vi "Edit Items.vi"(11 "Display State In":T1={"Persistent"={"Elements"=[], "PicElements"=[], "Limits"=[], "Selection"=[], "Selection Color"=0, "Highlight"=[], "Highlight Val"=0, "Highlight Color"={"Back"=0, "Edge"=0}, "Font"={"Details"={"Font Name:"="Lucida Sans", "Size"=24, "Strikeout?"=FALSE, "Italic?"=FALSE, "Underline?"=FALSE, "Outline?"=FALSE, "Shadow?"=FALSE, "Bold?"=TRUE}, "Color"=7697781}, "Bakground Color"=0}, "List Ref"=refnum, "nbVisible"=0, "FirstIdx"=0, "More.Width"=0}) -> (2 "Changed":bool, 3 "Display State out":T1={"Persistent"={"Elements"=[], "PicElements"=[], "Limits"=[], "Selection"=[], "Selection Color"=0, "Highlight"=[], "Highlight Val"=0, "Highlight Color"={"Back"=0, "Edge"=0}, "Font"={"Details"={"Font Name:"="Lucida Sans", "Size"=24, "Strikeout?"=FALSE, "Italic?"=FALSE, "Underline?"=FALSE, "Outline?"=FALSE, "Shadow?"=FALSE, "Bold?"=TRUE}, "Color"=7697781}, "Bakground Color"=0}, "List Ref"=refnum, "nbVisible"=0, "FirstIdx"=0, "More.Width"=0} caption="Display State Out")   [LabVIEW 2016, in "Horizontal MenuList.xctl"]
uses:
  Horizontal MenuList.xctl
  Horizontal MenuList_State.ctl
  Highlight Colors.ctl
  Edit_Actions.ctl
panel:
  out "Stop":bool
  in  "Move Down":bool
  in  "Move Up":bool
  in  "Delete":bool
  in  "Insert":bool
  out "Preview":picture
  in  "Item Pairs":i32(listbox)
  in  "Cancel":bool
  in  "OK":bool
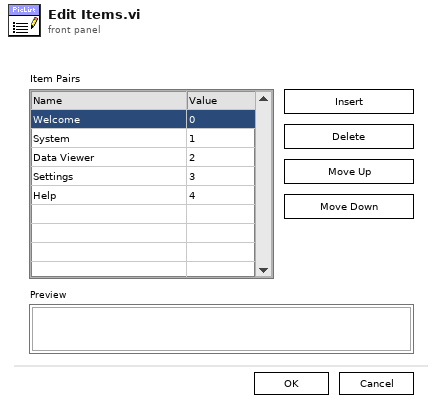
[diagram p1: front panel]
types:
  T1 = typedef "Horizontal MenuList.xctl/Horizontal MenuList_State.ctl" = cluster{"Persistent":cluster{"Elements":string[], "PicElements":picture[], "Limits":i32[], "Selection":picture[], "Selection Color":u32, "Highlight":picture[], "Highlight Val":i32, "Highlight Color":T2, "Font":cluster{"Details":cluster{"Font Name:":string, "Size":i16, "Strikeout?":bool, "Italic?":bool, "Underline?":bool, "Outline?":bool, "Shadow?":bool, "Bold?":bool}, "Color":u32}, "Bakground Color":u32}, "List Ref":refnum<vi>, "nbVisible":u8, "FirstIdx":u8, "More.Width":u8}
  T2 = typedef "Horizontal MenuList.xctl/Highlight Colors.ctl" = cluster{"Back":u32, "Edge":u32}
  T3 = typedef "Horizontal MenuList.xctl/Edit_Actions.ctl" = enum16{"Insert", "Delete", "Move Up", "Move Down"}
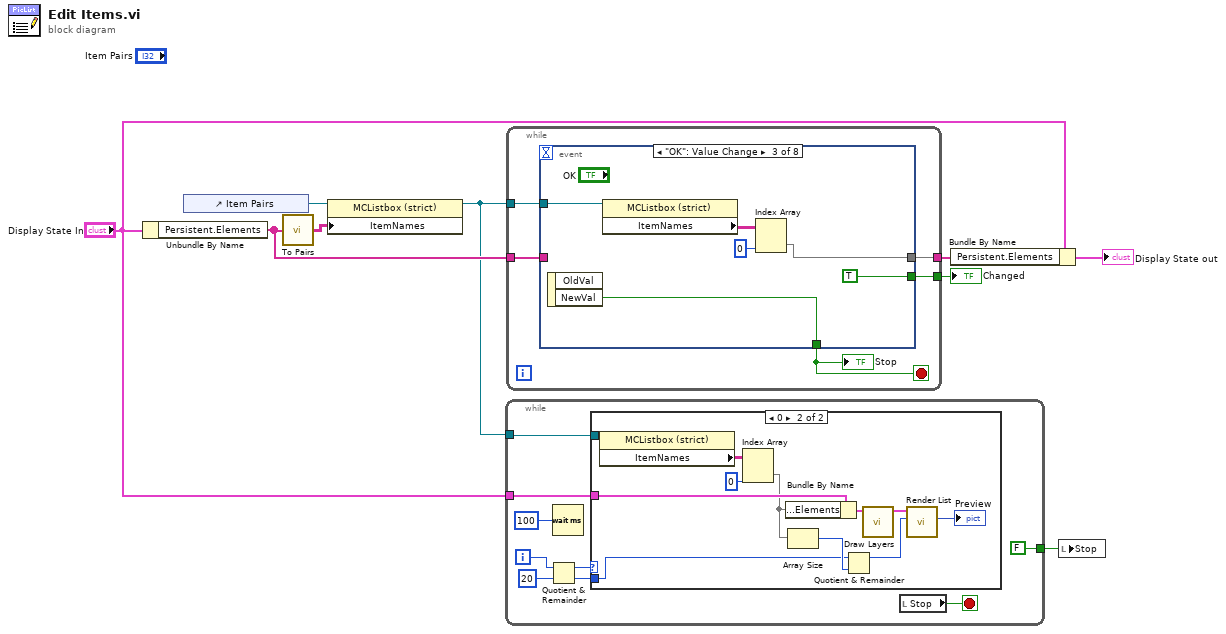
[diagram p0: block diagram]
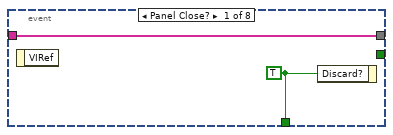
[diagram p3: hidden frame]
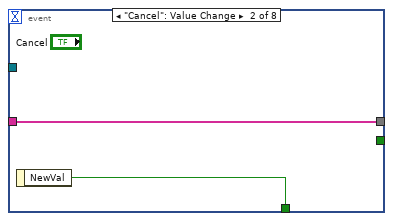
[diagram p4: hidden frame]
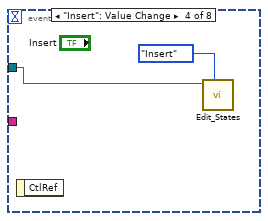
[diagram p5: hidden frame]
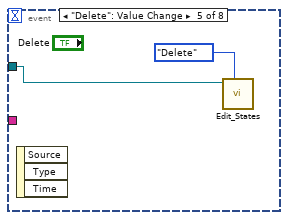
[diagram p6: hidden frame]
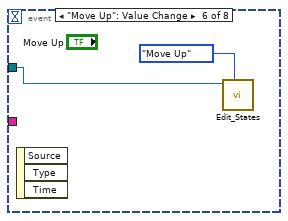
[diagram p7: hidden frame]
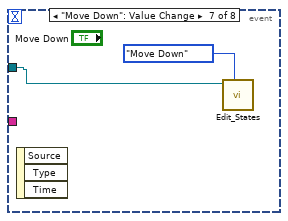
[diagram p8: hidden frame]
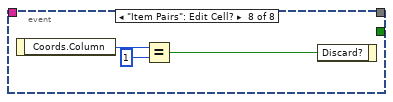
[diagram p9: hidden frame]
diagram:
  n1 = Unbundle By Name("Display State In") -> ("Persistent.Elements"=w6:string[])
  n2 = control-ref of="Item Pairs"() -> (w9:refnum<vi>)
  n3 = call "To Pairs.vi"("Elements"=w6) -> ("Array"=w5:string[][])  [unwired: 4 in]
  n4 = property class="MCListbox (strict)"(reference=w9, "ItemNames"=w5) -> (reference out=w3:refnum<vi>)  [unwired: 1 in, 1 out]
  n5 = while {
    tunnel: "Display State In" -> [w18]
    tunnel: w3 -> [w17]
    tunnel: [FALSE] -> w2
    i -> [w14]
    stop <- w16 stop-if-true
    n6 = Quotient & Remainder(x=w14, y=20) -> (x-y*floor(x/y)=w11:i32, floor(x/y)=w10:i32)
    n7 = Wait (ms)(milliseconds to wait=u32 100) -> ()  [unwired: 1 out]
    n8 = case shown="0" w11 {
      tunnel: w18 -> [_ w28]
      tunnel: w17 -> [_ w26]
      tunnel: w10 -> [_ w20]
      frame Default {
      }
      frame 0 {
        n9 = property class="MCListbox (strict)"(reference=w26) -> ("ItemNames"=w25:string[][])  [unwired: 1 in, 2 out]
        n10 = Index Array(array=w25, index (col)=0 ("disabled index (col)")) -> (element=w23:string[])  [unwired: 1 in]
        n11 = Bundle By Name(cluster=w28, "Persistent.Elements"=w23) -> (w29:T1)
        n12 = Array Size(array=w23) -> (size(s)=w22:i32)
        n13 = Quotient & Remainder(x=w20, y=w22) -> (x-y*floor(x/y)=w21:i32)  [unwired: 1 out]
        n14 = call "Draw Layers.vi"("Display State In in"=w29) -> ("Display State In out"=w27:T1)  [unwired: 10 in]
        n15 = call "Render List.vi"("Value"=w21, "Display State In"=w27) -> ("Selection"=→"Preview":picture)  [unwired: 6 in, 3 out]
      }
    }
    n16 = local read "Stop"() -> (w16:bool)
  }
  n17 = while {
    tunnel: w6 -> [w34]
    tunnel: w3 -> [w33]
    tunnel: [w32] -> w7
    tunnel: [w30] -> w1
    stop <- w31 stop-if-true
    n18 = event shown="[2] \"OK\": Value Change" {
      selector: _ -> [_ _ _ _ _ _ _ _]
      dyn-events: _ -> [_ _ _ _ _ _ _ _]
      timeout: _ -> [_ _ _ _ _ _ _ _]
      tunnel: [w36 w38 w44 _ _ _ _ _] -> w31
      tunnel: w34 -> [w35 w37 _ _ _ _ _ _]
      tunnel: w33 -> [_ _ w43 w46 w48 w50 w52 _]
      tunnel: [w35 w37 w40 _ _ _ _ _] -> w32
      tunnel: [_ _ TRUE _ _ _ _ _] -> w30
      event Panel Close? {
        w36 = TRUE ("Discard?")
        n19 = event-data() -> ()  [unwired: 1 in, 1 out]
        n20 = event-data("Discard?"=w36) -> ()  [unwired: 1 in, 1 out]
      }
      event "Cancel": Value Change {
        n21 = event-data() -> ("NewVal"=w38:bool)  [unwired: 1 in]
      }
      event "OK": Value Change {
        n22 = event-data() -> ("NewVal"=w44:bool)  [unwired: 1 in, 1 out]
        n23 = property class="MCListbox (strict)"(reference=w43) -> ("ItemNames"=w42:string[][])  [unwired: 1 in, 2 out]
        n24 = Index Array(array=w42, index (col)=0 ("disabled index (col)")) -> (element=w40:string[])  [unwired: 1 in]
      }
      event "Insert": Value Change {
        n25 = event-data() -> ()  [unwired: 1 in, 1 out]
        n26 = call "Edit_States.vi"("Action"=Edit_Actions."Insert", "MulticolumnListbox in"=w46) -> ()  [unwired: 9 in, 1 out]
      }
      event "Delete": Value Change {
        n27 = event-data() -> ()  [unwired: 1 in, 3 out]
        n28 = call "Edit_States.vi"("Action"=Edit_Actions."Delete", "MulticolumnListbox in"=w48) -> ()  [unwired: 9 in, 1 out]
      }
      event "Move Up": Value Change {
        n29 = event-data() -> ()  [unwired: 1 in, 3 out]
        n30 = call "Edit_States.vi"("Action"=Edit_Actions."Move Up", "MulticolumnListbox in"=w50) -> ()  [unwired: 9 in, 1 out]
      }
      event "Move Down": Value Change {
        n31 = event-data() -> ()  [unwired: 1 in, 3 out]
        n32 = call "Edit_States.vi"("Action"=Edit_Actions."Move Down", "MulticolumnListbox in"=w52) -> ()  [unwired: 9 in, 1 out]
      }
      event "Item Pairs": Edit Cell? {
        n33 = event-data() -> ("Coords.Column"=w55:i32)  [unwired: 1 in]
        n34 = Equal?(x=w55, y=1) -> (x = y?=w53:bool)
        n35 = event-data("Discard?"=w53) -> ()  [unwired: 1 in, 1 out]
      }
    }
    "Stop" <- w31
  }
  "Changed" <- w1
  n36 = Bundle By Name(cluster="Display State In", "Persistent.Elements"=w7) -> (→"Display State out":T1)
  n37 = local write "Stop"(w2) -> ()
